vi "CAN-SET.vi"(6 "DevIndex":u32, 9 "open?":bool, 10 "type":u32(ring)=2 items=["USB-CAN"=2, "USB-CAN2.0"=3]) -> (2 "success":bool, 3 "Param out":T2[](array[typedef]) {"ACR0" format="%x"})   [LabVIEW 2011]
uses:
  VIs/Param.ctl
  VIs/Baud rate Self Define.ctl
  VIs/ParamType.ctl
panel:
  in  "advance":bool
  in  "br_selfdef":T1={"BAUD"=0, "SJW"=1, "BRP"=1, "SAM"=0, "PHS2_SEL"=0, "SYN(nouse)"=1, "PRSEG"=1, "PHSEG1"=1, "PHSEG2"=1} {"PHSEG2" items=["CAN_BIT_1TQ"=1, "CAN_BIT_2TQ"=2, "CAN_BIT_3TQ"=3, "CAN_BIT_4TQ"=4, "CAN_BIT_5TQ"=5, "CAN_BIT_6TQ"=6, "CAN_BIT_7TQ"=7, "CAN_BIT_8TQ"=8]; "PHSEG1" items=["CAN_BIT_1TQ"=1, "CAN_BIT_2TQ"=2, "CAN_BIT_3TQ"=3, "CAN_BIT_4TQ"=4, "CAN_BIT_5TQ"=5, "CAN_BIT_6TQ"=6, "CAN_BIT_7TQ"=7, "CAN_BIT_8TQ"=8]; "PRSEG" items=["CAN_BIT_1TQ"=1, "CAN_BIT_2TQ"=2, "CAN_BIT_3TQ"=3, "CAN_BIT_4TQ"=4, "CAN_BIT_5TQ"=5, "CAN_BIT_6TQ"=6, "CAN_BIT_7TQ"=7, "CAN_BIT_8TQ"=8]; "PHS2_SEL" items=["由相位缓冲段1时间指定", "可编程"]; "SAM" items=["采样一次", "采样三次"]; "BRP" items=["1"=1, "2"=2, "3"=3, "4"=4, "5"=5, "6"=6, "7"=7, "8"=8, "9"=9, "10"=10, "11"=11, "12"=12, "13"=13, "14"=14, "15"=15, "16"=16, "17"=17, "18"=18, "19"=19, "20"=20, "21"=21, "22"=22, "23"=23, "24"=24, "25"=25, "26"=26, "27"=27, "28"=28, "29"=29, "30"=30, "31"=31, "32"=32, "33"=33, "34"=34, "35"=35, "36"=36, "37"=37, "38"=38, "39"=39, "40"=40, "41"=41, "42"=42, "43"=43, "44"=44, "45"=45, "46"=46, "47"=47, "48"=48, "49"=49, "50"=50, "51"=51, "52"=52, "53"=53, "54"=54, "55"=55, "56"=56, "57"=57, "58"=58, "59"=59, "60"=60, "61"=61, "62"=62, "63"=63, "64"=64]; "SJW" items=["1TQ"=1, "2TQ"=2, "3TQ"=3, "4TQ"=4]; "SYN(nouse)" items=["CAN_BIT_1TQ"=1]}
  in  "Filter":u8(ring)=1 caption="滤波方式：" items=["接收所有类型"=1, "只收标准帧"=2, "只收扩展帧"=3]
  in  "set2":bool
  in  "set1":bool
  in  "channel":enum16{"通道1", "通道2"}(ring) caption="CAN通道"
  in  "屏蔽码":u32=4294967295 caption="过滤屏蔽码:" format="%08x"
  in  "验收码":u32=2147483648 caption="过滤验收码:" format="%08x"
  in  "工作模式":u16(ring) items=["正常工作", "仅监帧听模式", "自测模试（环回模式）"]
  in  "set0":bool
  in  "br":u32(ring)=8 caption="波特率:" items=["Self Define", "5k bps", "10k bps", "20k bps", "40k bps", "50k bps", "80k bps", "100k bps", "125k bps", "200k bps", "250k bps", "400k bps", "500k bps", "666k bps", "800k bps", "1000k bps", "33.33k bps", "66.66k bps", "83.33k bps"]
  # "注：CAN波特率=16000000/(同步段+传播时间段+相位缓冲段1+相位缓冲段2)/预分频"
  # "波特率设置"
  # "工作模式"
  # "滤波器"
  # "(HEX)"
  # "(HEX)"
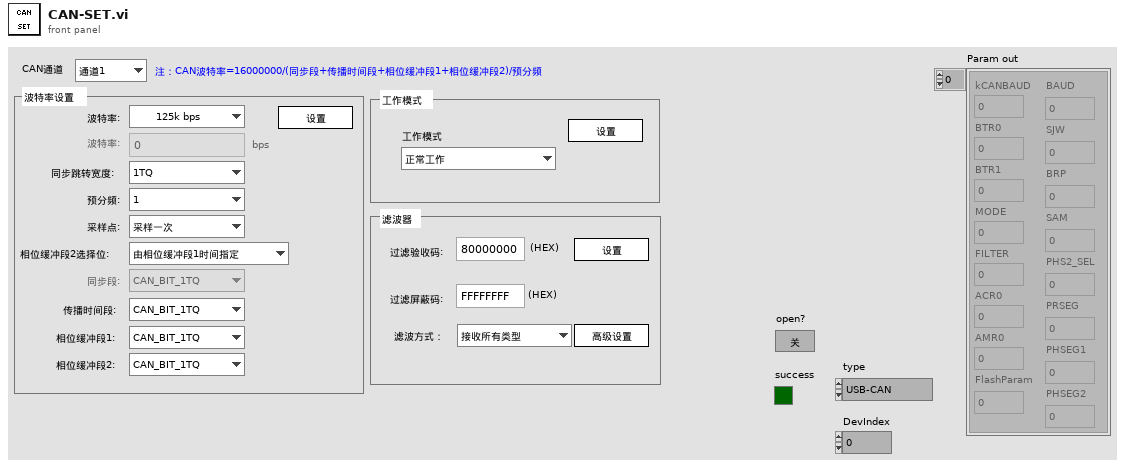
[diagram p1: front panel]
types:
  T1 = typedef "Baud rate Self Define.ctl" = cluster{"BAUD":u32, "SJW":u8, "BRP":u8, "SAM":u8, "PHS2_SEL":u8, "SYN(nouse)":u8, "PRSEG":u8, "PHSEG1":u8, "PHSEG2":u8}
  T2 = typedef "Param.ctl" = cluster{"kCANBAUD":u8, "BTR0":u8, "BTR1":u8, "MODE":u8, "FILTER":u8, "ACR0":u32, "AMR0":u32, "FlashParam":u32, "BAUD":u32, "SJW":u8, "BRP":u8, "SAM":u8, "PHS2_SEL":u8, "PRSEG":u8, "PHSEG1":u8, "PHSEG2":u8}
  T3 = enum8{"Enabled", "Disabled", "Disabled and Grayed Out"}
  T4 = typedef "ParamType.ctl" = u32
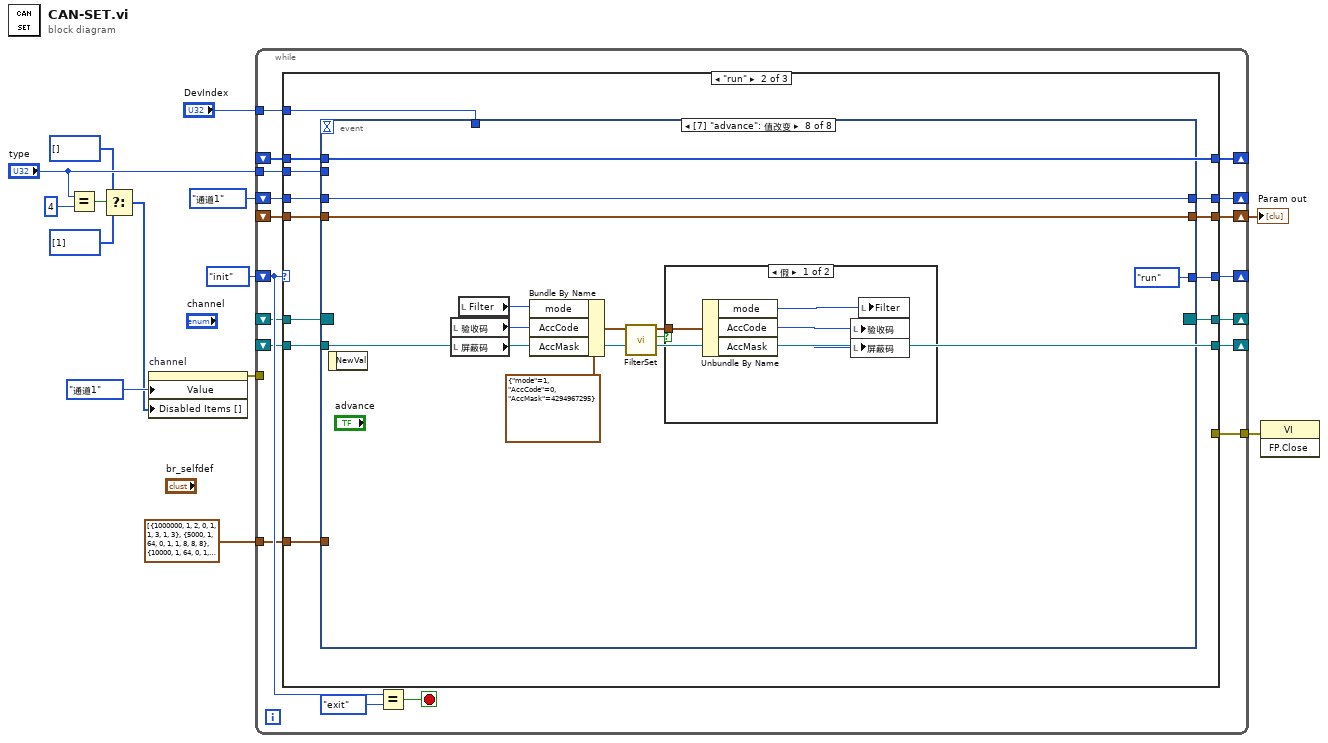
[diagram p0: block diagram]
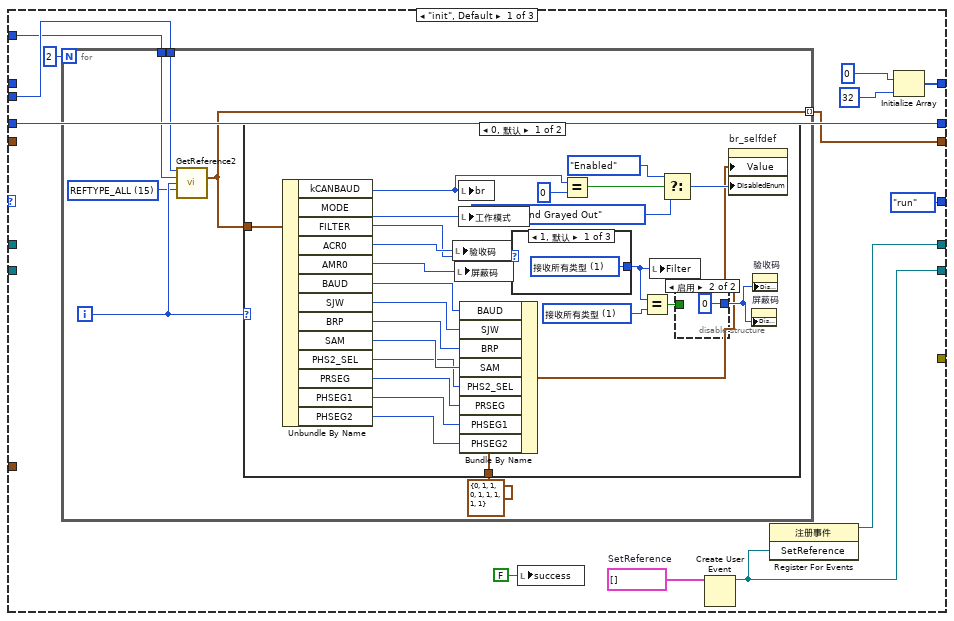
[diagram p2: hidden frame]
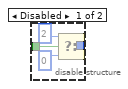
[diagram p3: hidden frame]
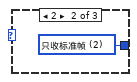
[diagram p4: hidden frame]
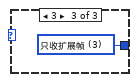
[diagram p5: hidden frame]
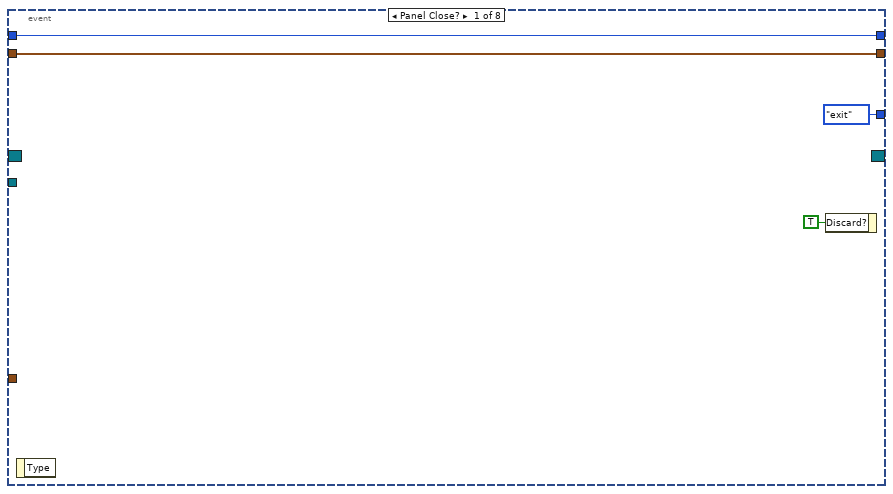
[diagram p7: hidden frame]
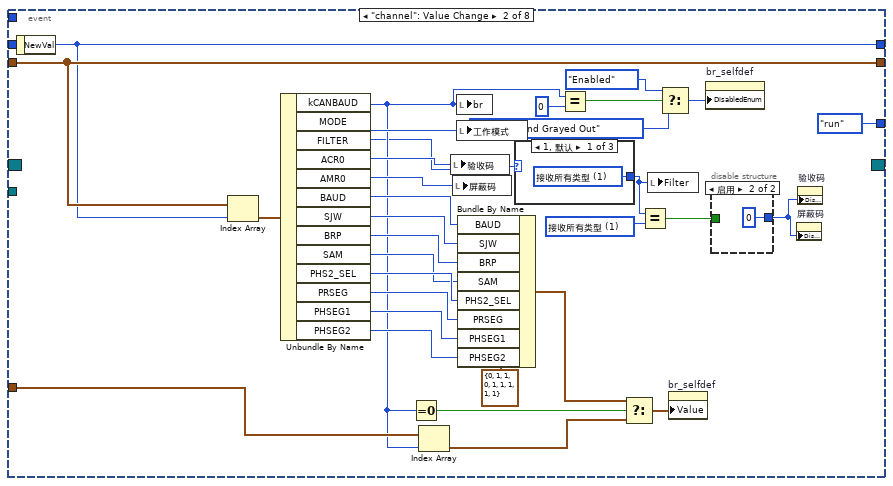
[diagram p8: hidden frame]
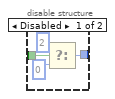
[diagram p9: hidden frame]
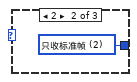
[diagram p10: hidden frame]
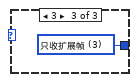
[diagram p11: hidden frame]
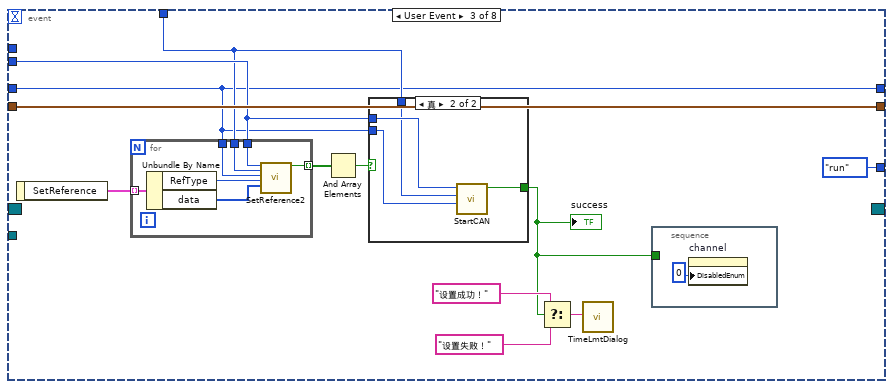
[diagram p12: hidden frame]
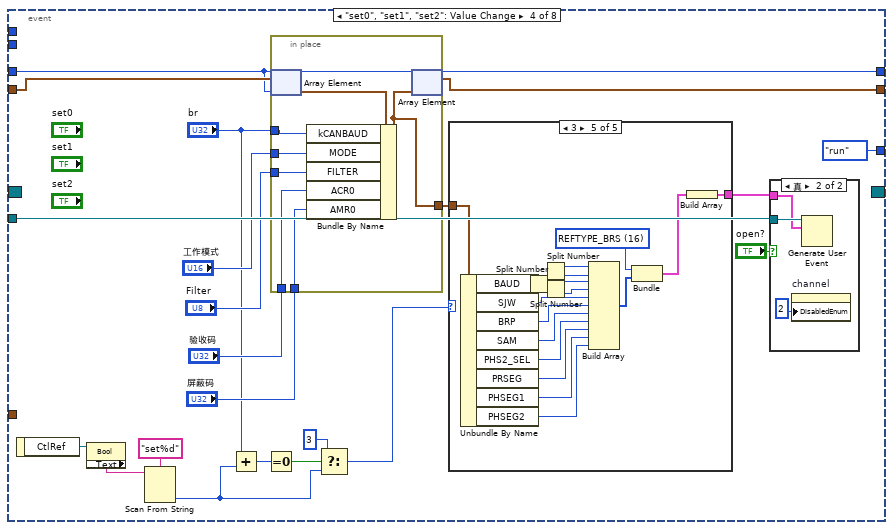
[diagram p14: hidden frame]
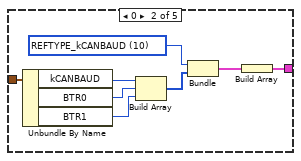
[diagram p16: hidden frame]
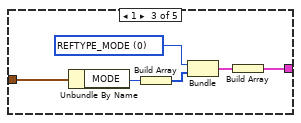
[diagram p17: hidden frame]
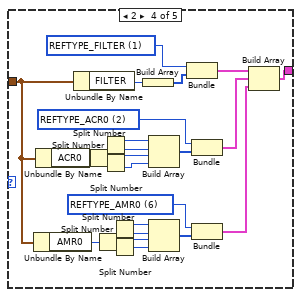
[diagram p18: hidden frame]
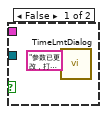
[diagram p19: hidden frame]
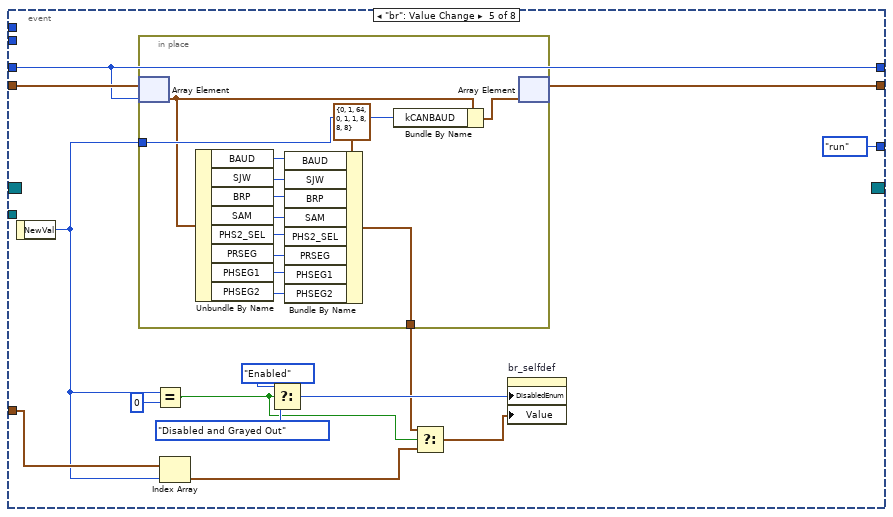
[diagram p20: hidden frame]
diagram:
  n1 = Equal?(x="type", y=u32 4) -> (x = y?=w7:bool)
  n2 = Select(t=i32[] [] ("禁用项[]"), s=w7, f=i32[] [1] ("禁用项[]")) -> (s? t:f=w5:i32[])
  n3 = property on="channel" class="Enum (严格)"("Value"=enum16{"通道1", "通道2"}."通道1" ("channel"), "Disabled Items []"=w5) -> (error out=w12:errorcluster)  [unwired: 2 in, 1 out]
  n4 = while {
    shift-right: [w31] -> w2
    shift-left: _ -> [w32]
    shift-right: [w30] -> _
    shift-left: enum16{"init", "run", "exit"}."init" -> [w29]
    tunnel: [w26] -> w13
    shift-right: [w25] -> _
    shift-left: _ -> [w23]
    shift-right: [w24] -> _
    shift-left: _ -> [w22]
    tunnel: "type" -> [w21]
    shift-right: [w20] -> _
    shift-left: _ -> [w19]
    tunnel: "DevIndex" -> [w18]
    shift-right: [w16] -> _
    shift-left: enum16{"通道1", "通道2"}."通道1" ("NewVal") -> [w17]
    tunnel: w12 -> [_]
    tunnel: T1[] [{"BAUD"=1000000, "SJW"=1, "BRP"=2, "SAM"=0, "PHS2_SEL"=1, "SYN(nouse)"=1, "PRSEG"=3, "PHSEG1"=1, "PHSEG2"=3}, {"BAUD"=5000, "SJW"=1, "BRP"=64, "SAM"=0, "PHS2_SEL"=1, "SYN(nouse)"=1, "PRSEG"=8, "PHSEG1"=8, "PHSEG2"=8}, {"BAUD"=10000, "SJW"=1, "BRP"=64, "SAM"=0, "PHS2_SEL"=1, "SYN(nouse)"=1, "PRSEG"=8, "PHSEG1"=8, "PHSEG2"=8}, {"BAUD"=20000, "SJW"=1, "BRP"=50, "SAM"=0, "PHS2_SEL"=1, "SYN(nouse)"=1, "PRSEG"=5, "PHSEG1"=5, "PHSEG2"=5}, {"BAUD"=40000, "SJW"=1, "BRP"=16, "SAM"=0, "PHS2_SEL"=1, "SYN(nouse)"=1, "PRSEG"=8, "PHSEG1"=8, "PHSEG2"=8}, {"BAUD"=50000, "SJW"=1, "BRP"=20, "SAM"=0, "PHS2_SEL"=1, "SYN(nouse)"=1, "PRSEG"=5, "PHSEG1"=5, "PHSEG2"=5}, {"BAUD"=80000, "SJW"=1, "BRP"=8, "SAM"=0, "PHS2_SEL"=1, "SYN(nouse)"=1, "PRSEG"=8, "PHSEG1"=8, "PHSEG2"=8}, {"BAUD"=100000, "SJW"=1, "BRP"=10, "SAM"=0, "PHS2_SEL"=1, "SYN(nouse)"=1, "PRSEG"=7, "PHSEG1"=4, "PHSEG2"=4}, {"BAUD"=125000, "SJW"=1, "BRP"=8, "SAM"=0, "PHS2_SEL"=1, "SYN(nouse)"=1, "PRSEG"=7, "PHSEG1"=4, "PHSEG2"=4}, {"BAUD"=200000, "SJW"=1, "BRP"=4, "SAM"=0, "PHS2_SEL"=1, "SYN(nouse)"=1, "PRSEG"=7, "PHSEG1"=6, "PHSEG2"=6}, {"BAUD"=250000, "SJW"=1, "BRP"=4, "SAM"=0, "PHS2_SEL"=1, "SYN(nouse)"=1, "PRSEG"=7, "PHSEG1"=4, "PHSEG2"=4}, {"BAUD"=400000, "SJW"=1, "BRP"=2, "SAM"=0, "PHS2_SEL"=1, "SYN(nouse)"=1, "PRSEG"=7, "PHSEG1"=6, "PHSEG2"=6}, {"BAUD"=500000, "SJW"=1, "BRP"=2, "SAM"=0, "PHS2_SEL"=1, "SYN(nouse)"=1, "PRSEG"=7, "PHSEG1"=4, "PHSEG2"=4}, {"BAUD"=666000, "SJW"=1, "BRP"=2, "SAM"=0, "PHS2_SEL"=1, "SYN(nouse)"=1, "PRSEG"=3, "PHSEG1"=4, "PHSEG2"=4}, {"BAUD"=800000, "SJW"=1, "BRP"=2, "SAM"=0, "PHS2_SEL"=1, "SYN(nouse)"=1, "PRSEG"=3, "PHSEG1"=3, "PHSEG2"=3}, {"BAUD"=1000000, "SJW"=1, "BRP"=2, "SAM"=0, "PHS2_SEL"=1, "SYN(nouse)"=1, "PRSEG"=3, "PHSEG1"=1, "PHSEG2"=3}, {"BAUD"=33333, "SJW"=1, "BRP"=32, "SAM"=0, "PHS2_SEL"=1, "SYN(nouse)"=1, "PRSEG"=4, "PHSEG1"=5, "PHSEG2"=5}, {"BAUD"=66666, "SJW"=1, "BRP"=16, "SAM"=0, "PHS2_SEL"=1, "SYN(nouse)"=1, "PRSEG"=4, "PHSEG1"=5, "PHSEG2"=5}, {"BAUD"=83333, "SJW"=1, "BRP"=8, "SAM"=0, "PHS2_SEL"=1, "SYN(nouse)"=1, "PRSEG"=7, "PHSEG1"=8, "PHSEG2"=8}] -> [w15]
    stop <- w27 stop-if-true
    n5 = case shown="\"run\"" w29 {
      tunnel: w32 -> [_ w96 w362]
      tunnel: [w35 w95 w362] -> w31
      tunnel: [enum16{"init", "run", "exit"}."run" w94 enum16{"init", "run", "exit"}."exit"] -> w30
      tunnel: [_ _ errorcluster {"status"=FALSE, "code"=0, "source"=""} ("错误输入（无错误）")] -> w26
      tunnel: [w44 w89 _] -> w25
      tunnel: [w43 w90 _] -> w24
      tunnel: w23 -> [_ w93 w359]
      tunnel: w22 -> [_ w90 w357]
      tunnel: w21 -> [w34 w92 _]
      tunnel: [w40 w91 _] -> w20
      tunnel: w19 -> [_ w91 _]
      tunnel: w18 -> [w33 w88 _]
      tunnel: w17 -> [w37 w87 w356]
      tunnel: [w37 w86 w356] -> w16
      tunnel: w15 -> [_ w85 _]
      frame "init", Default {
        w38 = cluster{"RefType":u32, "data":u8[]}[] []  # SetReference
        n6 = for {
          N: 2 -> [_]
          tunnel: [w46] -> w35 mode=indexing
          tunnel: w34 -> [w50]
          tunnel: w33 -> [w49]
          i -> [w51]
          w48 = T4 15 items=["REFTYPE_MODE"=0, "REFTYPE_FILTER"=1, "REFTYPE_ACR0"=2, "REFTYPE_AMR0"=6, "REFTYPE_kCANBAUD"=10, "REFTYPE_CANRX_EN"=13, "REFTYPE_UARTBAUD"=14, "REFTYPE_ALL"=15, "REFTYPE_BRS"=16] ("RefType")
          n7 = call "GetReference2.vi"("DeviceType"=w50, "DeviceInd"=w49, "CANInd"=w51, "RefType"=w48) -> ("Param"=w46:T2)  [unwired: 9 in, 2 out]
          n8 = case shown="0, 默认" w51 {
            tunnel: w46 -> [w70 _]
            tunnel: T1 {"BAUD"=0, "SJW"=1, "BRP"=1, "SAM"=0, "PHS2_SEL"=1, "SYN(nouse)"=1, "PRSEG"=1, "PHSEG1"=1, "PHSEG2"=1} ("br_selfdef") -> [w67 _]
            frame 0, Default {
              w53 = u8 1 items=["接收所有类型"=1, "只收标准帧"=2, "只收扩展帧"=3] ("Filter")
              n9 = Unbundle By Name(w70) -> ("kCANBAUD"=w56:u8, "MODE"=w76:u8, "FILTER"=w54:u8, "ACR0"=w75:u32, "AMR0"=w74:u32, "BAUD"=w65:u32, "SJW"=w64:u8, "BRP"=w63:u8, "SAM"=w62:u8, "PHS2_SEL"=w61:u8, "PRSEG"=w60:u8, "PHSEG1"=w59:u8, "PHSEG2"=w58:u8)
              n10 = local write "验收码"(w75) -> ()
              n11 = local write "屏蔽码"(w74) -> ()
              n12 = local write "br"(w56) -> ()
              n13 = local write "工作模式"(w76) -> ()
              n14 = Bundle By Name(cluster=w67, "BAUD"=w65, "SJW"=w64, "BRP"=w63, "SAM"=w62, "PHS2_SEL"=w61, "PRSEG"=w60, "PHSEG1"=w59, "PHSEG2"=w58) -> (w55:T1)
              n15 = case shown="1, 默认" w54 {
                tunnel: [w82 w83 w84] -> w52
                frame 1, Default {
                  w82 = u8 1 items=["接收所有类型"=1, "只收标准帧"=2, "只收扩展帧"=3] ("Filter")
                }
                frame 2 {
                  w83 = u8 2 items=["接收所有类型"=1, "只收标准帧"=2, "只收扩展帧"=3] ("Filter")
                }
                frame 3 {
                  w84 = u8 3 items=["接收所有类型"=1, "只收标准帧"=2, "只收扩展帧"=3] ("Filter")
                }
              }
              n16 = Equal?(x=w56, y=u32 0) -> (x = y?=w57:bool)
              n17 = Equal?(x=w52, y=w53) -> (x = y?=w69:bool)
              n18 = local write "Filter"(w52) -> ()
              n19 = Select(t=T3."Enabled" ("禁用"), s=w57, f=T3."Disabled and Grayed Out") -> (s? t:f=w66:T3)
              n20 = disable-structure shown="启用" {
                disable-tunnel: w69 -> [w80 _]
                disable-tunnel: [w79 0] -> w68
                frame Disabled {
                  n21 = Select(t=2, s=w80, f=0) -> (s? t:f=w79:i32)
                }
                frame Enabled {
                }
              }
              n22 = property on="br_selfdef" class="Clust (严格)"("Value"=w55, "DisabledEnum"=w66) -> ()  [unwired: 2 in, 2 out]
              n23 = property on="屏蔽码" class="DigNum (严格)"("DisabledEnum"=w68) -> ()  [unwired: 2 in, 2 out]
              n24 = property on="验收码" class="DigNum (严格)"("DisabledEnum"=w68) -> ()  [unwired: 2 in, 2 out]
            }
            frame 1 {
            }
          }
        }
        n25 = local write "success"(FALSE ("success")) -> ()
        n26 = Create User Event(user event datatype=w38) -> (user event=w43:refnum<user-event>)  [unwired: 1 in, 1 out]
        n27 = register-events(w43) -> (reference out=w44:refnum<event-registration>)  [unwired: 2 in, 1 out]
        n28 = Initialize Array(u8 0, 32 ("维数大小")) -> (w40:u8[])
      }
      frame "run" {
        n29 = event shown="[7] \"advance\": 值改变" {
          selector: w93 -> [_ _ _ _ _ _ _ _]
          dyn-events: [_ _ _ _ _ _ _ _] -> w89
          timeout: _ -> [_ _ _ _ _ _ _ _]
          tunnel: w96 -> [w99 w131 w152 w175 w265 w294 w315 w347]
          tunnel: [w99 w131 w152 w173 w264 w292 w313 w347] -> w95
          tunnel: [enum16{"init", "run", "exit"}."exit" enum16{"init", "run", "exit"}."run" enum16{"init", "run", "exit"}."run" enum16{"init", "run", "exit"}."run" enum16{"init", "run", "exit"}."run" enum16{"init", "run", "exit"}."run" enum16{"init", "run", "exit"}."run" enum16{"init", "run", "exit"}."run"] -> w94
          tunnel: w90 -> [_ _ _ w184 _ _ _ _]
          tunnel: w92 -> [_ _ w146 _ _ _ _ _]
          tunnel: w91 -> [_ _ _ _ _ _ _ _]
          tunnel: w88 -> [_ _ w145 _ _ _ _ _]
          tunnel: w87 -> [w97 _ w142 w174 w259 w293 w314 w350]
          tunnel: [w97 w130 w142 w174 w259 w293 w314 w350] -> w86
          tunnel: w85 -> [_ w106 _ _ w260 _ _ _]
          event Panel Close? {
            n30 = event-data() -> ()  [unwired: 1 in, 1 out]
            n31 = event-data("Discard?"=TRUE ("放弃？")) -> ()  [unwired: 1 in, 1 out]
          }
          event "channel": Value Change {
            w101 = u8 1 items=["接收所有类型"=1, "只收标准帧"=2, "只收扩展帧"=3] ("Filter")
            n32 = event-data() -> ("NewVal"=w130:enum16{"通道1", "通道2"})  [unwired: 1 in]
            n33 = Index Array(array=w131, index=w130) -> (element=w110:T2)
            n34 = Unbundle By Name(w110) -> ("kCANBAUD"=w105:u8, "MODE"=w112:u8, "FILTER"=w103:u8, "ACR0"=w113:u32, "AMR0"=w114:u32, "BAUD"=w121:u32, "SJW"=w122:u8, "BRP"=w123:u8, "SAM"=w124:u8, "PHS2_SEL"=w125:u8, "PRSEG"=w126:u8, "PHSEG1"=w127:u8, "PHSEG2"=w128:u8)
            n35 = Equal To 0?(x=w105) -> (x = 0?=w109:bool)
            n36 = Index Array(array=w106, index=w105) -> (element=w104:T1)
            n37 = local write "验收码"(w113) -> ()
            n38 = local write "屏蔽码"(w114) -> ()
            n39 = local write "br"(w105) -> ()
            n40 = local write "工作模式"(w112) -> ()
            n41 = Bundle By Name(cluster=T1 {"BAUD"=0, "SJW"=1, "BRP"=1, "SAM"=0, "PHS2_SEL"=1, "SYN(nouse)"=1, "PRSEG"=1, "PHSEG1"=1, "PHSEG2"=1} ("br_selfdef"), "BAUD"=w121, "SJW"=w122, "BRP"=w123, "SAM"=w124, "PHS2_SEL"=w125, "PRSEG"=w126, "PHSEG1"=w127, "PHSEG2"=w128) -> (w108:T1)
            n42 = case shown="1, 默认" w103 {
              tunnel: [w138 w139 w140] -> w102
              frame 1, Default {
                w138 = u8 1 items=["接收所有类型"=1, "只收标准帧"=2, "只收扩展帧"=3] ("Filter")
              }
              frame 2 {
                w139 = u8 2 items=["接收所有类型"=1, "只收标准帧"=2, "只收扩展帧"=3] ("Filter")
              }
              frame 3 {
                w140 = u8 3 items=["接收所有类型"=1, "只收标准帧"=2, "只收扩展帧"=3] ("Filter")
              }
            }
            n43 = Equal?(x=w105, y=u32 0) -> (x = y?=w129:bool)
            n44 = Select(t=w108, s=w109, f=w104) -> (s? t:f=w107:T1)
            n45 = Equal?(x=w102, y=w101) -> (x = y?=w118:bool)
            n46 = local write "Filter"(w102) -> ()
            n47 = Select(t=T3."Enabled" ("禁用"), s=w129, f=T3."Disabled and Grayed Out") -> (s? t:f=w120:T3)
            n48 = property on="br_selfdef" class="Clust (严格)"("Value"=w107) -> ()  [unwired: 2 in, 2 out]
            n49 = property on="br_selfdef" class="Clust (严格)"("DisabledEnum"=w120) -> ()  [unwired: 2 in, 2 out]
            n50 = disable-structure shown="启用" {
              disable-tunnel: [w134 0] -> w119
              disable-tunnel: w118 -> [w133 _]
              frame Disabled {
                n51 = Select(t=2, s=w133, f=0) -> (s? t:f=w134:i32)
              }
              frame Enabled {
              }
            }
            n52 = property on="屏蔽码" class="DigNum (严格)"("DisabledEnum"=w119) -> ()  [unwired: 2 in, 2 out]
            n53 = property on="验收码" class="DigNum (严格)"("DisabledEnum"=w119) -> ()  [unwired: 2 in, 2 out]
          }
          event User Event {
            n54 = event-data() -> ("SetReference"=w144:cluster{"RefType":u32, "data":u8[]}[])  [unwired: 1 in]
            n55 = for {
              tunnel: [w160] -> w147 mode=indexing
              tunnel: w146 -> [w159]
              tunnel: w145 -> [w158]
              tunnel: w142 -> [w157]
              tunnel: w144 -> [w156] mode=indexing
              n56 = Unbundle By Name(w156) -> ("RefType"=w155:u32, "data"=w154:u8[])
              n57 = call "SetReference2.vi"("DeviceType"=w159, "DeviceInd"=w158, "CANInd"=w157, "RefType"=w155, "pData"=w154) -> ("Success"=w160:bool)  [unwired: 13 in, 1 out]
            }
            n58 = And Array Elements(Boolean array=w147) -> (logical AND=w143:bool)
            n59 = case shown="真" w143 {
              tunnel: w146 -> [_ w164]
              tunnel: w142 -> [_ w162]
              tunnel: [_ w161] -> w141
              tunnel: w145 -> [_ w163]
              frame False {
              }
              frame True {
                n60 = call "StartCAN.vi"("CANInd"=w162, "DeciceInd"=w163, "DeviceType"=w164) -> ("Valid"=w161:bool)  [unwired: 7 in, 1 out]
              }
            }
            "success" <- w141
            n61 = Select(t="设置成功！", s=w141, f="设置失败！") -> (s? t:f=w148:string)
            n62 = call "TimeLmtDialog.vi"("Infoin"=w148) -> ()  [unwired: 11 in]
            n63 = stacked-sequence {
              tunnel: w141 -> [_]
              frame #0 {
                n64 = property on="channel" class="Enum (严格)"("DisabledEnum"=0) -> ()  [unwired: 2 in, 2 out]
              }
            }
          }
          event "set0", "set1", "set2": Value Change {
            n65 = event-data() -> ("CtlRef"=w179:refnum<vi>)  [unwired: 1 in]
            n66 = property class="Bool"(reference=w179) -> ("Label.Text"=w178:string)  [unwired: 1 in, 2 out]
            n67 = Scan From String(format string="set%d" ("格式字符串"), input string=w178) -> (output 1=w168:i32)  [unwired: 3 in, 3 out]
            n68 = Add(x="br", y=w168) -> (x+y=w166:u32)
            n69 = Equal To 0?(x=w166) -> (x = 0?=w165:bool)
            n70 = in-place {
              in-place-border: "br" -> [w192]
              in-place-border: "工作模式" -> [w191]
              in-place-border: "验收码" -> [w190]
              in-place-border: "屏蔽码" -> [w189]
              in-place-border: [w187] -> w172
              in-place-border: "Filter" -> [w186]
              n71 = in-place-array #1(w175, w174) -> (w188:T2)
              n72 = Bundle By Name(cluster=w188, "kCANBAUD"=w192, "MODE"=w191, "FILTER"=w186, "ACR0"=w190, "AMR0"=w189) -> (w187:T2)
              n73 = in-place-array #1(w187) -> (w173:T2[])  [unwired: 1 out]
            }
            n74 = Select(t=3, s=w165, f=w168) -> (s? t:f=w169:i32)
            n75 = case shown="3" w169 {
              tunnel: w172 -> [_ w200 w206 w214 w243]
              tunnel: [_ w194 w202 w210 w242] -> w176
              frame -1, Default {
              }
              frame 0 {
                w193 = T4 10 items=["REFTYPE_MODE"=0, "REFTYPE_FILTER"=1, "REFTYPE_ACR0"=2, "REFTYPE_AMR0"=6, "REFTYPE_kCANBAUD"=10, "REFTYPE_CANRX_EN"=13, "REFTYPE_UARTBAUD"=14, "REFTYPE_ALL"=15, "REFTYPE_BRS"=16] ("RefType")
                n76 = Unbundle By Name(w200) -> ("kCANBAUD"=w199:u8, "BTR0"=w198:u8, "BTR1"=w197:u8)
                n77 = Build Array(w199, w198, w197) -> (w196:u8[])
                n78 = Bundle("RefType"=w193, w196) -> (w195:cluster{"RefType":T4, u8[]})  [unwired: 1 in]
                n79 = Build Array(w195) -> (w194:cluster{"RefType":T4, u8[]}[])
              }
              frame 1 {
                w201 = T4 0 items=["REFTYPE_MODE"=0, "REFTYPE_FILTER"=1, "REFTYPE_ACR0"=2, "REFTYPE_AMR0"=6, "REFTYPE_kCANBAUD"=10, "REFTYPE_CANRX_EN"=13, "REFTYPE_UARTBAUD"=14, "REFTYPE_ALL"=15, "REFTYPE_BRS"=16] ("RefType")
                n80 = Unbundle By Name(w206) -> ("MODE"=w205:u8)
                n81 = Build Array(w205) -> (w204:u8[])
                n82 = Bundle("RefType"=w201, w204) -> (w203:cluster{"RefType":T4, u8[]})  [unwired: 1 in]
                n83 = Build Array(w203) -> (w202:cluster{"RefType":T4, u8[]}[])
              }
              frame 2 {
                w207 = T4 6 items=["REFTYPE_MODE"=0, "REFTYPE_FILTER"=1, "REFTYPE_ACR0"=2, "REFTYPE_AMR0"=6, "REFTYPE_kCANBAUD"=10, "REFTYPE_CANRX_EN"=13, "REFTYPE_UARTBAUD"=14, "REFTYPE_ALL"=15, "REFTYPE_BRS"=16] ("RefType")
                w208 = T4 2 items=["REFTYPE_MODE"=0, "REFTYPE_FILTER"=1, "REFTYPE_ACR0"=2, "REFTYPE_AMR0"=6, "REFTYPE_kCANBAUD"=10, "REFTYPE_CANRX_EN"=13, "REFTYPE_UARTBAUD"=14, "REFTYPE_ALL"=15, "REFTYPE_BRS"=16] ("RefType")
                w209 = T4 1 items=["REFTYPE_MODE"=0, "REFTYPE_FILTER"=1, "REFTYPE_ACR0"=2, "REFTYPE_AMR0"=6, "REFTYPE_kCANBAUD"=10, "REFTYPE_CANRX_EN"=13, "REFTYPE_UARTBAUD"=14, "REFTYPE_ALL"=15, "REFTYPE_BRS"=16] ("RefType")
                n84 = Unbundle By Name(w214) -> ("AMR0"=w216:u32)
                n85 = Unbundle By Name(w214) -> ("ACR0"=w229:u32)
                n86 = Unbundle By Name(w214) -> ("FILTER"=w232:u8)
                n87 = Split Number(x=w229) -> (hi(x)=w228:u16, lo(x)=w227:u16)
                n88 = Split Number(x=w216) -> (hi(x)=w217:u16, lo(x)=w218:u16)
                n89 = Split Number(x=w228) -> (hi(x)=w226:u8, lo(x)=w225:u8)
                n90 = Split Number(x=w227) -> (hi(x)=w224:u8, lo(x)=w223:u8)
                n91 = Split Number(x=w217) -> (hi(x)=w219:u8, lo(x)=w220:u8)
                n92 = Split Number(x=w218) -> (hi(x)=w221:u8, lo(x)=w222:u8)
                n93 = Build Array(w232) -> (w231:u8[])
                n94 = Build Array(w226, w225, w224, w223) -> (w230:u8[])
                n95 = Build Array(w219, w220, w221, w222) -> (w215:u8[])
                n96 = Bundle("RefType"=w209, w231) -> (w213:cluster{"RefType":T4, u8[]})  [unwired: 1 in]
                n97 = Bundle("RefType"=w208, w230) -> (w212:cluster{"RefType":T4, u8[]})  [unwired: 1 in]
                n98 = Bundle("RefType"=w207, w215) -> (w211:cluster{"RefType":T4, u8[]})  [unwired: 1 in]
                n99 = Build Array(w213, w212, w211) -> (w210:cluster{"RefType":T4, u8[]}[])
              }
              frame 3 {
                w240 = T4 16 items=["REFTYPE_MODE"=0, "REFTYPE_FILTER"=1, "REFTYPE_ACR0"=2, "REFTYPE_AMR0"=6, "REFTYPE_kCANBAUD"=10, "REFTYPE_CANRX_EN"=13, "REFTYPE_UARTBAUD"=14, "REFTYPE_ALL"=15, "REFTYPE_BRS"=16] ("RefType")
                n100 = Unbundle By Name(w243) -> ("BAUD"=w250:u32, "SJW"=w239:u8, "BRP"=w238:u8, "SAM"=w237:u8, "PHS2_SEL"=w236:u8, "PRSEG"=w235:u8, "PHSEG1"=w234:u8, "PHSEG2"=w233:u8)
                n101 = Split Number(x=w250) -> (hi(x)=w249:u16, lo(x)=w248:u16)
                n102 = Split Number(x=w249) -> (hi(x)=w247:u8, lo(x)=w246:u8)
                n103 = Split Number(x=w248) -> (hi(x)=w245:u8, lo(x)=w244:u8)
                n104 = Build Array(w247, w246, w245, w244, w239, w238, w237, w236, w235, w234, w233) -> (w251:u8[])
                n105 = Bundle("RefType"=w240, w251) -> (w241:cluster{"RefType":T4, u8[]})  [unwired: 1 in]
                n106 = Build Array(w241) -> (w242:cluster{"RefType":T4, u8[]}[])
              }
            }
            n107 = case shown="真" "open?" {
              tunnel: w184 -> [_ w255]
              tunnel: w176 -> [_ w254]
              frame False {
                n108 = call "TimeLmtDialog.vi"("Infoin"="参数已更改，打开设备生效！") -> ()  [unwired: 11 in]
              }
              frame True {
                n109 = property on="channel" class="Enum (严格)"("DisabledEnum"=2) -> ()  [unwired: 2 in, 2 out]
                n110 = Generate User Event(user event=w255, event data cluster=w254) -> ()  [unwired: 1 in, 2 out]
              }
            }
          }
          event "br": Value Change {
            n111 = event-data() -> ("NewVal"=w256:u32)  [unwired: 1 in]
            n112 = in-place {
              in-place-border: w256 -> [w282]
              in-place-border: [w270] -> w261
              n113 = in-place-array #2(w265, w259) -> (w280:T2)
              n114 = Unbundle By Name(w280) -> ("BAUD"=w271:u32, "SJW"=w272:u8, "BRP"=w273:u8, "SAM"=w274:u8, "PHS2_SEL"=w275:u8, "PRSEG"=w276:u8, "PHSEG1"=w277:u8, "PHSEG2"=w278:u8)
              n115 = Bundle By Name(cluster=T1 {"BAUD"=0, "SJW"=1, "BRP"=64, "SAM"=0, "PHS2_SEL"=1, "SYN(nouse)"=1, "PRSEG"=8, "PHSEG1"=8, "PHSEG2"=8} ("br_selfdef"), "BAUD"=w271, "SJW"=w272, "BRP"=w273, "SAM"=w274, "PHS2_SEL"=w275, "PRSEG"=w276, "PHSEG1"=w277, "PHSEG2"=w278) -> (w270:T1)
              n116 = Bundle By Name(cluster=w280, "kCANBAUD"=w282) -> (w281:T2)
              n117 = in-place-array #2(w281) -> (w264:T2[])  [unwired: 1 out]
            }
            n118 = Equal?(x=w256, y=u32 0) -> (x = y?=w262:bool)
            n119 = Index Array(array=w260, index=w256) -> (element=w258:T1)
            n120 = Select(t=T3."Enabled" ("禁用"), s=w262, f=T3."Disabled and Grayed Out") -> (s? t:f=w263:T3)
            n121 = Select(t=w261, s=w262, f=w258) -> (s? t:f=w257:T1)
            n122 = property on="br_selfdef" class="Clust (严格)"("DisabledEnum"=w263, "Value"=w257) -> ()  [unwired: 2 in, 2 out]
          }
          event Value Change {
            # "注：CAN波特率=16000000/(同步段+传播时间段+相位缓冲段1+相位缓冲段2)/预分频"
            n123 = event-data() -> ("NewVal.BRP"=w297:u8, "NewVal.SYN(nouse)"=w299:u8, "NewVal.PRSEG"=w286:u8, "NewVal.PHSEG1"=w283:u8, "NewVal.PHSEG2"=w285:u8, "NewVal"=w290:T1, "NewVal.PHS2_SEL"=w289:u8)  [unwired: 1 in]
            n124 = Equal?(x=w289, y=u8 0) -> (x = y?=w287:bool)
            n125 = Select(t=w283, s=w287, f=w285) -> (s? t:f=w284:u8)
            n126 = property on="PHSEG2" class="Ring (严格)"("Value"=w284) -> ()  [unwired: 2 in, 2 out]
            n127 = Compound Arithmetic op=ADD(w299, w286, w283, w284) -> (w295:u8)
            n128 = Divide(x=16000000.0, y=w297) -> (x/y=w296:dbl)
            n129 = Divide(x=w296, y=w295) -> (x/y=w291:dbl)
            n130 = property on="BAUD" class="DigNum (严格)"("Value"=w291) -> ()  [unwired: 2 in, 2 out]
            n131 = in-place {
              in-place-border: w291 -> [w309]
              in-place-border: w290 -> [w308]
              n132 = in-place-array #3(w294, w293) -> (w311:T2)
              n133 = Unbundle By Name(w308) -> ("SJW"=w301:u8, "BRP"=w302:u8, "SAM"=w303:u8, "PHS2_SEL"=w304:u8, "PRSEG"=w305:u8, "PHSEG1"=w306:u8, "PHSEG2"=w307:u8)
              n134 = Bundle By Name(cluster=w311, "BAUD"=w309, "SJW"=w301, "BRP"=w302, "SAM"=w303, "PHS2_SEL"=w304, "PRSEG"=w305, "PHSEG1"=w306, "PHSEG2"=w307) -> (w310:T2)
              n135 = in-place-array #3(w310) -> (w292:T2[])  [unwired: 1 out]
            }
          }
          event "Filter": Value Change {
            n136 = event-data() -> ("NewVal"=w312:u8)  [unwired: 1 in]
            n137 = in-place {
              in-place-border: w312 -> [w324]
              w325 = u8 1 items=["接收所有类型"=1, "只收标准帧"=2, "只收扩展帧"=3] ("Filter")
              n138 = in-place-array #4(w315, w314) -> (w321:T2)
              n139 = case shown="3" w324 {
                tunnel: [w339 w340 w341] -> w322
                frame 1, Default {
                  w339 = u8 1 items=["接收所有类型"=1, "只收标准帧"=2, "只收扩展帧"=3] ("Filter")
                }
                frame 2 {
                  w340 = u8 2 items=["接收所有类型"=1, "只收标准帧"=2, "只收扩展帧"=3] ("Filter")
                }
                frame 3 {
                  w341 = u8 3 items=["接收所有类型"=1, "只收标准帧"=2, "只收扩展帧"=3] ("Filter")
                }
              }
              n140 = Unbundle By Name(w321) -> ("ACR0"=w320:u32, "AMR0"=w319:u32)
              n141 = Equal?(x=w322, y=w325) -> (x = y?=w326:bool)
              n142 = local write "Filter"(w322) -> ()
              n143 = disable-structure shown="启用" {
                disable-tunnel: w326 -> [w335 _]
                disable-tunnel: w320 -> [w330 w338]
                disable-tunnel: w319 -> [w329 w337]
                disable-tunnel: [w328 w338] -> w318
                disable-tunnel: [w327 w337] -> w317
                frame Disabled {
                  n144 = Select(t=0, s=w335, f=0) -> (s? t:f=w331:i32)
                  n145 = Select(t=u32 0, s=w335, f=w330) -> (s? t:f=w328:u32)
                  n146 = Select(t=u32 4294967295, s=w335, f=w329) -> (s? t:f=w327:u32)
                  n147 = property on="屏蔽码" class="DigNum (严格)"("DisabledEnum"=w331, "Value"=w327) -> ()  [unwired: 2 in, 2 out]
                  n148 = property on="验收码" class="DigNum (严格)"("DisabledEnum"=w331, "Value"=w328) -> ()  [unwired: 2 in, 2 out]
                }
                frame Enabled {
                }
              }
              n149 = Bundle By Name(cluster=w321, "FILTER"=w322, "ACR0"=w318, "AMR0"=w317) -> (w323:T2)
              n150 = in-place-array #4(w323) -> (w313:T2[])  [unwired: 1 out]
            }
          }
          event "advance": Value Change {
            n151 = event-data() -> ()  [unwired: 1 in, 1 out]
            n152 = local read "验收码"() -> (w345:u32)
            n153 = local read "屏蔽码"() -> (w344:u32)
            n154 = local read "Filter"() -> (w346:u8)
            n155 = Bundle By Name(cluster=cluster{"mode":u8, "AccCode":u32, "AccMask":u32} {"mode"=1, "AccCode"=0, "AccMask"=4294967295} ("ParamIn"), "mode"=w346, "AccCode"=w345, "AccMask"=w344) -> (w348:cluster{"mode":u8, "AccCode":u32, "AccMask":u32})
            n156 = call "FilterSet.vi"("ParamIn"=w348) -> ("Cancel？"=w343:bool, "ParamOut"=w342:cluster{"mode":u8, "AccCode":u32, "AccMask":u32})  [unwired: 8 in, 1 out]
            n157 = case shown="假" w343 {
              tunnel: w342 -> [w355 _]
              frame False {
                n158 = Unbundle By Name(w355) -> ("mode"=w354:u8, "AccCode"=w353:u32, "AccMask"=w352:u32)
                n159 = local write "验收码"(w353) -> ()
                n160 = local write "屏蔽码"(w352) -> ()
                n161 = local write "Filter"(w354) -> ()
              }
              frame True {
              }
            }
          }
        }
      }
      frame "exit" {
        n162 = Unregister For Events(event registration refnum=w359) -> (error out=w358:errorcluster)  [unwired: 1 in]
        n163 = Destroy User Event(user event=w357, error in=w358) -> ()  [unwired: 1 out]
      }
    }
    n164 = Equal?(x=w29, y=enum16{"init", "run", "exit"}."exit") -> (x = y?=w27:bool)
  }
  "Param out" <- w2
  n165 = invoke class="VI" method="FP.Close"(error in=w13) -> ()  [unwired: 2 in, 3 out]
